vi "Read Value at Path.vi"   [LabVIEW 2020, in "Variant Data Manipulation.lvlib"]
uses:
  Variant Data Manipulation.lvlib
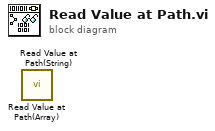
[diagram p0: block diagram]
diagram:
  n1 = call "Read Value at Path(Array).vi"() -> ()  [unwired: 9 in, 3 out]
  n2 = call "Read Value at Path(String).vi"() -> ()  [unwired: 9 in, 3 out]
